vi "VrmVISACheckResponse.vi"(8 "error in (no error)":errorcluster, 10 "Response":string) -> (0 "error out":errorcluster, 2 "Response out":string)   [LabVIEW 2025, in "MyTriton.lvlib"]
uses:
  MyTriton.lvlib
  <vilib>/regexp/Match Regular Expression.xnode
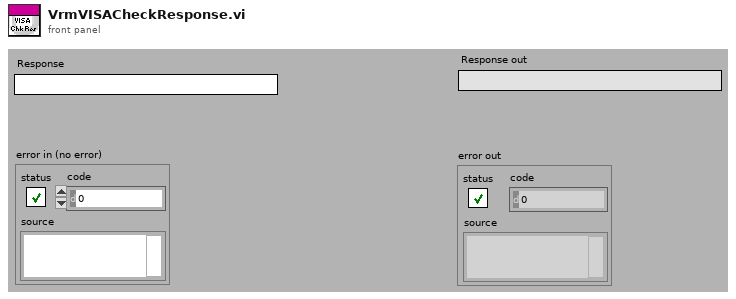
[diagram p1: front panel]
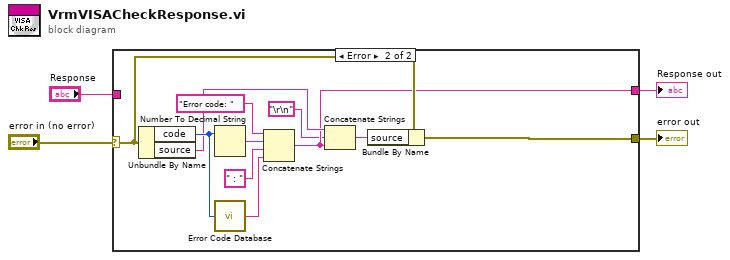
[diagram p0: block diagram]
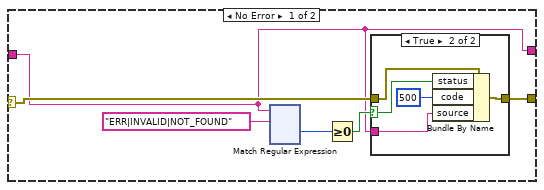
[diagram p2: hidden frame]
diagram:
  n1 = case shown="Error" "error in (no error)" {
    selector: "error in (no error)" -> [w8 w140]
    tunnel: "Response" -> [w5 _]
    tunnel: [w9 w136] -> w2
    tunnel: [w5 w138] -> w1
    frame No Error {
      n2 = xnode "Match Regular Expression"("input string"=w5, "regular expression"="ERR|INVALID|NOT_FOUND") -> ("offset past match"=w7:i32)  [unwired: 4 in, 4 out]
      n3 = Greater Or Equal To 0?(x=w7) -> (x >= 0?=w6:bool)
      n4 = case shown="True" w6 {
        selector: w6 -> [_ w14]
        tunnel: [w11 w16] -> w9
        tunnel: w8 -> [w11 w15]
        tunnel: w5 -> [_ w12]
        frame False {
        }
        frame True {
          n5 = Bundle By Name(cluster=w15, "status"=w14, "code"=500, "source"=w12) -> (w16:errorcluster)
        }
      }
    }
    frame Error {
      n6 = Unbundle By Name(w140) -> ("code"=w144:i32, "source"=w139:string)
      n7 = Number To Decimal String(number=w144) -> (decimal integer string=w143:string)  [unwired: 1 in]
      n8 = call <vilib>:"Error Code Database.vi"("Error Code"=w144) -> ("Error Text"=w141:string)
      n9 = Concatenate Strings("Error code: " ("string"), w143, " : " ("string"), w141) -> (w138:string)
      n10 = Concatenate Strings(w139, "\r\n", w138) -> (w137:string)
      n11 = Bundle By Name(cluster=w140, "source"=w137) -> (w136:errorcluster)
    }
  }
  "Response out" <- w1
  "error out" <- w2
